vi "WriteCommands.vi"(8 "error in (no error)":errorcluster, 9 "timeout in ms (100)":i32=100, 10 "Multi-line String":string, 11 "IO Queue":refnum<queue>) -> (0 "error out":errorcluster, 1 "timed out?":bool)   [LabVIEW 2020, in "TextControlledInstrum.lvlib"]
uses:
  TextControlledInstrum.lvlib
  IOQueuePacket.ctl
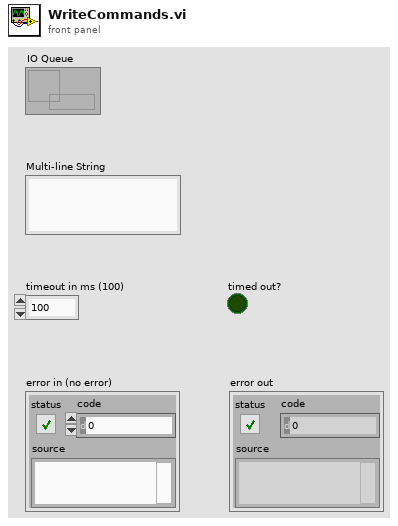
[diagram p1: front panel]
types:
  T1 = typedef "TextControlledInstrum.lvlib/IOQueuePacket.ctl" = cluster{"Operation":enum16{"read", "write", "reserved2", "reserved3", "reserved4", "reserved5", "reserved6", "reserved7"}, "Data":string, "Queue":refnum<queue>}
  T2 = enum16{"read", "write", "reserved2", "reserved3", "reserved4", "reserved5", "reserved6", "reserved7"}
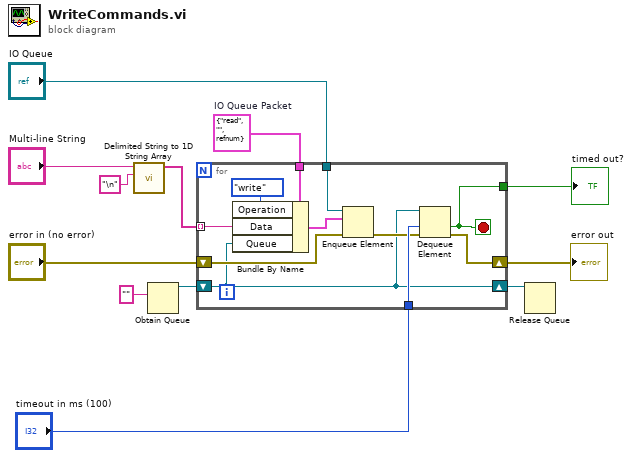
[diagram p0: block diagram]
diagram:
  w6 = T1 {"Operation"=enum."read", "Data"="", "Queue"=refnum}  # IO Queue Packet
  n1 = call <vilib>:"Delimited String to 1D String Array.vi"("delimiter"="\n", "delimited string"="Multi-line String") -> ("string array"=w12:string[])  [unwired: 9 in]
  n2 = Obtain Queue(element data type="") -> (queue out=w3:refnum<queue>)  [unwired: 4 in, 2 out]
  n3 = for {
    shift-right: [w15] -> w9
    shift-left: "error in (no error)" -> [w22]
    tunnel: "IO Queue" -> [w20]
    tunnel: w12 -> [w19] mode=indexing
    tunnel: w6 -> [w18]
    tunnel: "timeout in ms (100)" -> [w17]
    tunnel: [w14] -> w2
    shift-right: [w13] -> w1
    shift-left: w3 -> [w13]
    stop <- w14 stop-if-true
    n4 = Bundle By Name(cluster=w18, "Operation"=T2."write", "Data"=w19, "Queue"=w13) -> (w23:T1)
    n5 = Enqueue Element(queue=w20, element=w23, error in (no error)=w22) -> (error out=w16:errorcluster)  [unwired: 1 in, 2 out]
    n6 = Dequeue Element(queue=w13, timeout in ms (-1)=w17, error in (no error)=w16) -> (timed out?=w14:bool, error out=w15:errorcluster)  [unwired: 2 out]
  }
  "error out" <- w9
  "timed out?" <- w2
  n7 = Release Queue(queue=w1) -> ()  [unwired: 2 in, 3 out]
